vi "数据库保存子vi.vi"(0 "#1 Pressure":string, 1 "Part No.":string, 2 "Result":string, 3 "#2 Leakage":string, 4 "2D Code":string, 6 "Person":string, 8 "#2 Pressure":string, 9 "#1 Leakage":string, 10 "Serial No.":string, 11 "Time":string) -> ()   [LabVIEW 2014]
panel:
  out "error out":errorcluster
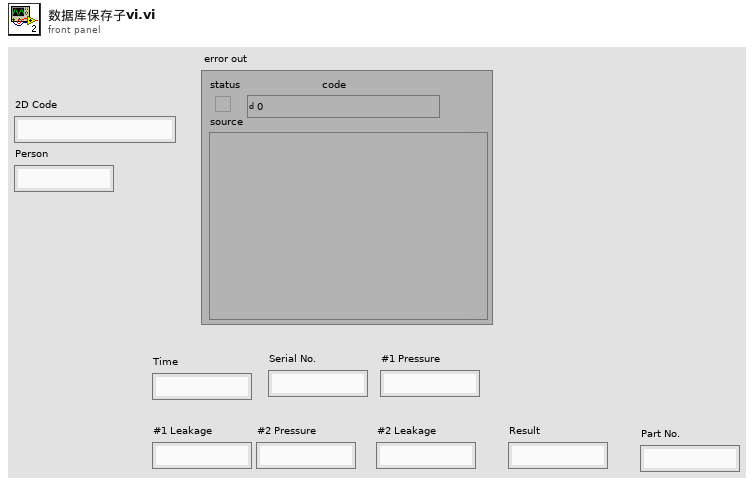
[diagram p1: front panel]
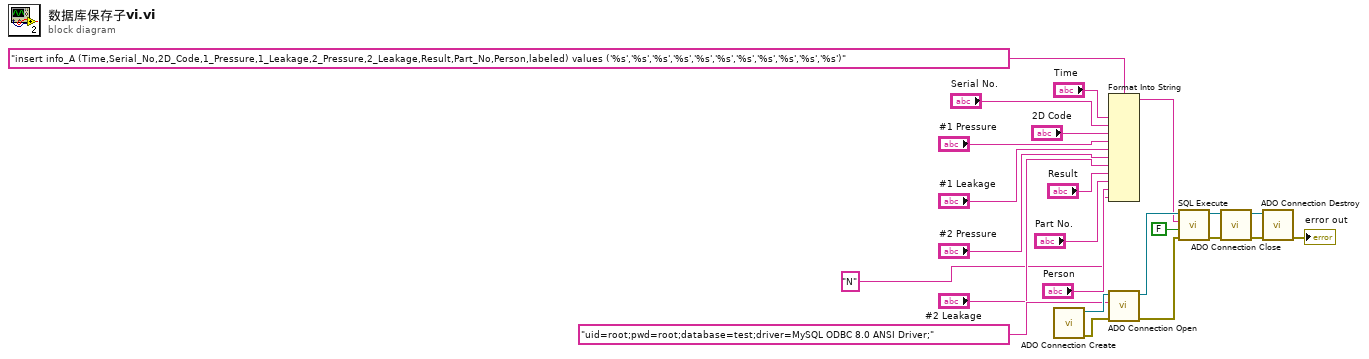
[diagram p0: block diagram]
diagram:
  n1 = call "ADO Connection Create.vi"() -> ("error out"=w23:errorcluster, "ADODB._Connection Out"=w24:refnum<k7>)  [unwired: 10 in]
  n2 = Format Into String(format string="insert info_A (Time,Serial_No,2D_Code,1_Pressure,1_Leakage,2_Pressure,2_Leakage,Result,Part_No,Person,labeled) values ('%s','%s','%s','%s','%s','%s','%s','%s','%s','%s','%s')" ("Command Text"), "Time", "Serial No.", "2D Code", "#1 Pressure", "#1 Leakage", "#2 Pressure", "#2 Leakage", "Result", "Part No.", "Person", "N") -> (resulting string=w10:string)  [unwired: 2 in, 1 out]
  n3 = call "ADO Connection Open.vi"("error in (no error)"=w23, "ConnectionString"="uid=root;pwd=root;database=test;driver=MySQL ODBC 8.0 ANSI Driver;", "ADODB._Connection In"=w24) -> ("error out"=w21:errorcluster, "ADODB._Connection Out"=w22:refnum<k7>)  [unwired: 7 in]
  n4 = call "SQL Execute.vi"("error in (no error)"=w21, "Return Data (T)"=FALSE, "Command Text"=w10, "ADODB._Connection In"=w22) -> ("error out"=w19:errorcluster, "ADODB._Connection Out"=w20:refnum<k7>)  [unwired: 4 in, 2 out]
  n5 = call "ADO Connection Close.vi"("error in (no error)"=w19, "ADODB._Connection In"=w20) -> ("error out"=w17:errorcluster, "ADODB._Connection Out"=w18:refnum<k7>)  [unwired: 8 in]
  n6 = call "ADO Connection Destroy.vi"("error in (no error)"=w17, "ADODB._Connection In"=w18) -> ("error out"=→"error out":errorcluster)  [unwired: 9 in]
